vi "ProcessingVehiclesCommandString.vi"(11 "input string":string) -> (3 "output cluster":T1)   [LabVIEW 2013]
panel:
  out "Lane Offset":dbl
  out "Vehicle Id":i32
  out "Time":dbl
  out "Current Distance":dbl
  out "Desired Distance":dbl
  out "Velocity Value":dbl format="%#_13g"
  out "Is Cruise Control":bool
  out "Lane String":string
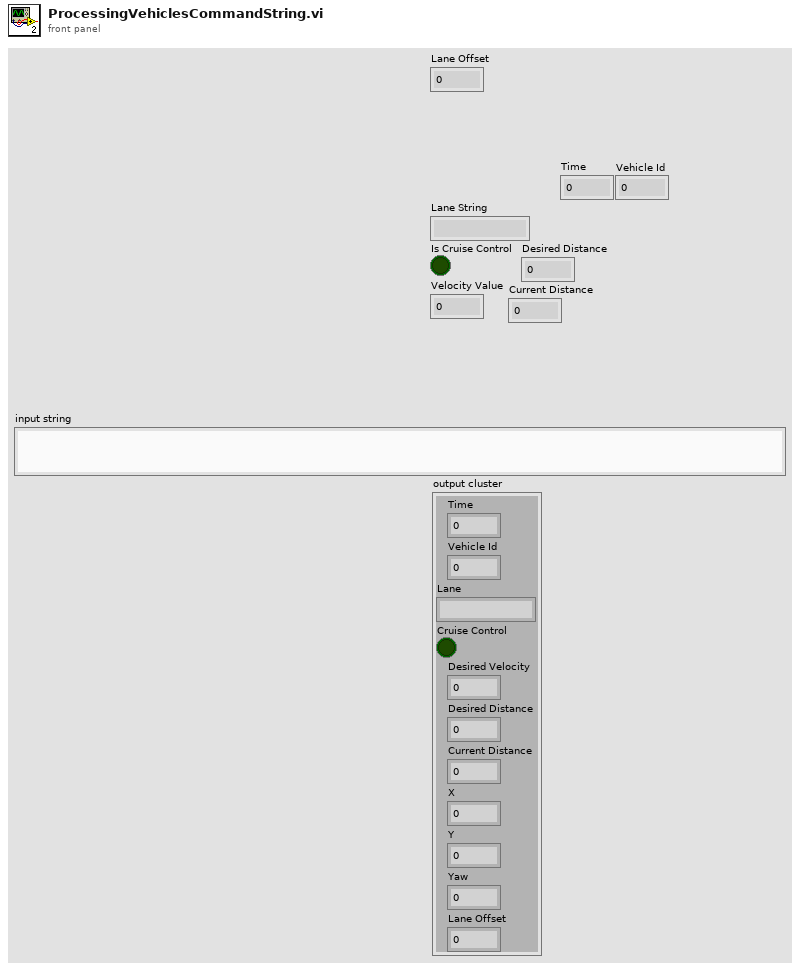
[diagram p1: front panel]
types:
  T1 = cluster{"Time":dbl, "Vehicle Id":i32, "Lane":string, "Cruise Control":bool, "Desired Velocity":dbl, "Desired Distance":dbl, "Current Distance":dbl, "X":dbl, "Y":dbl, "Yaw":dbl, "Lane Offset":dbl}
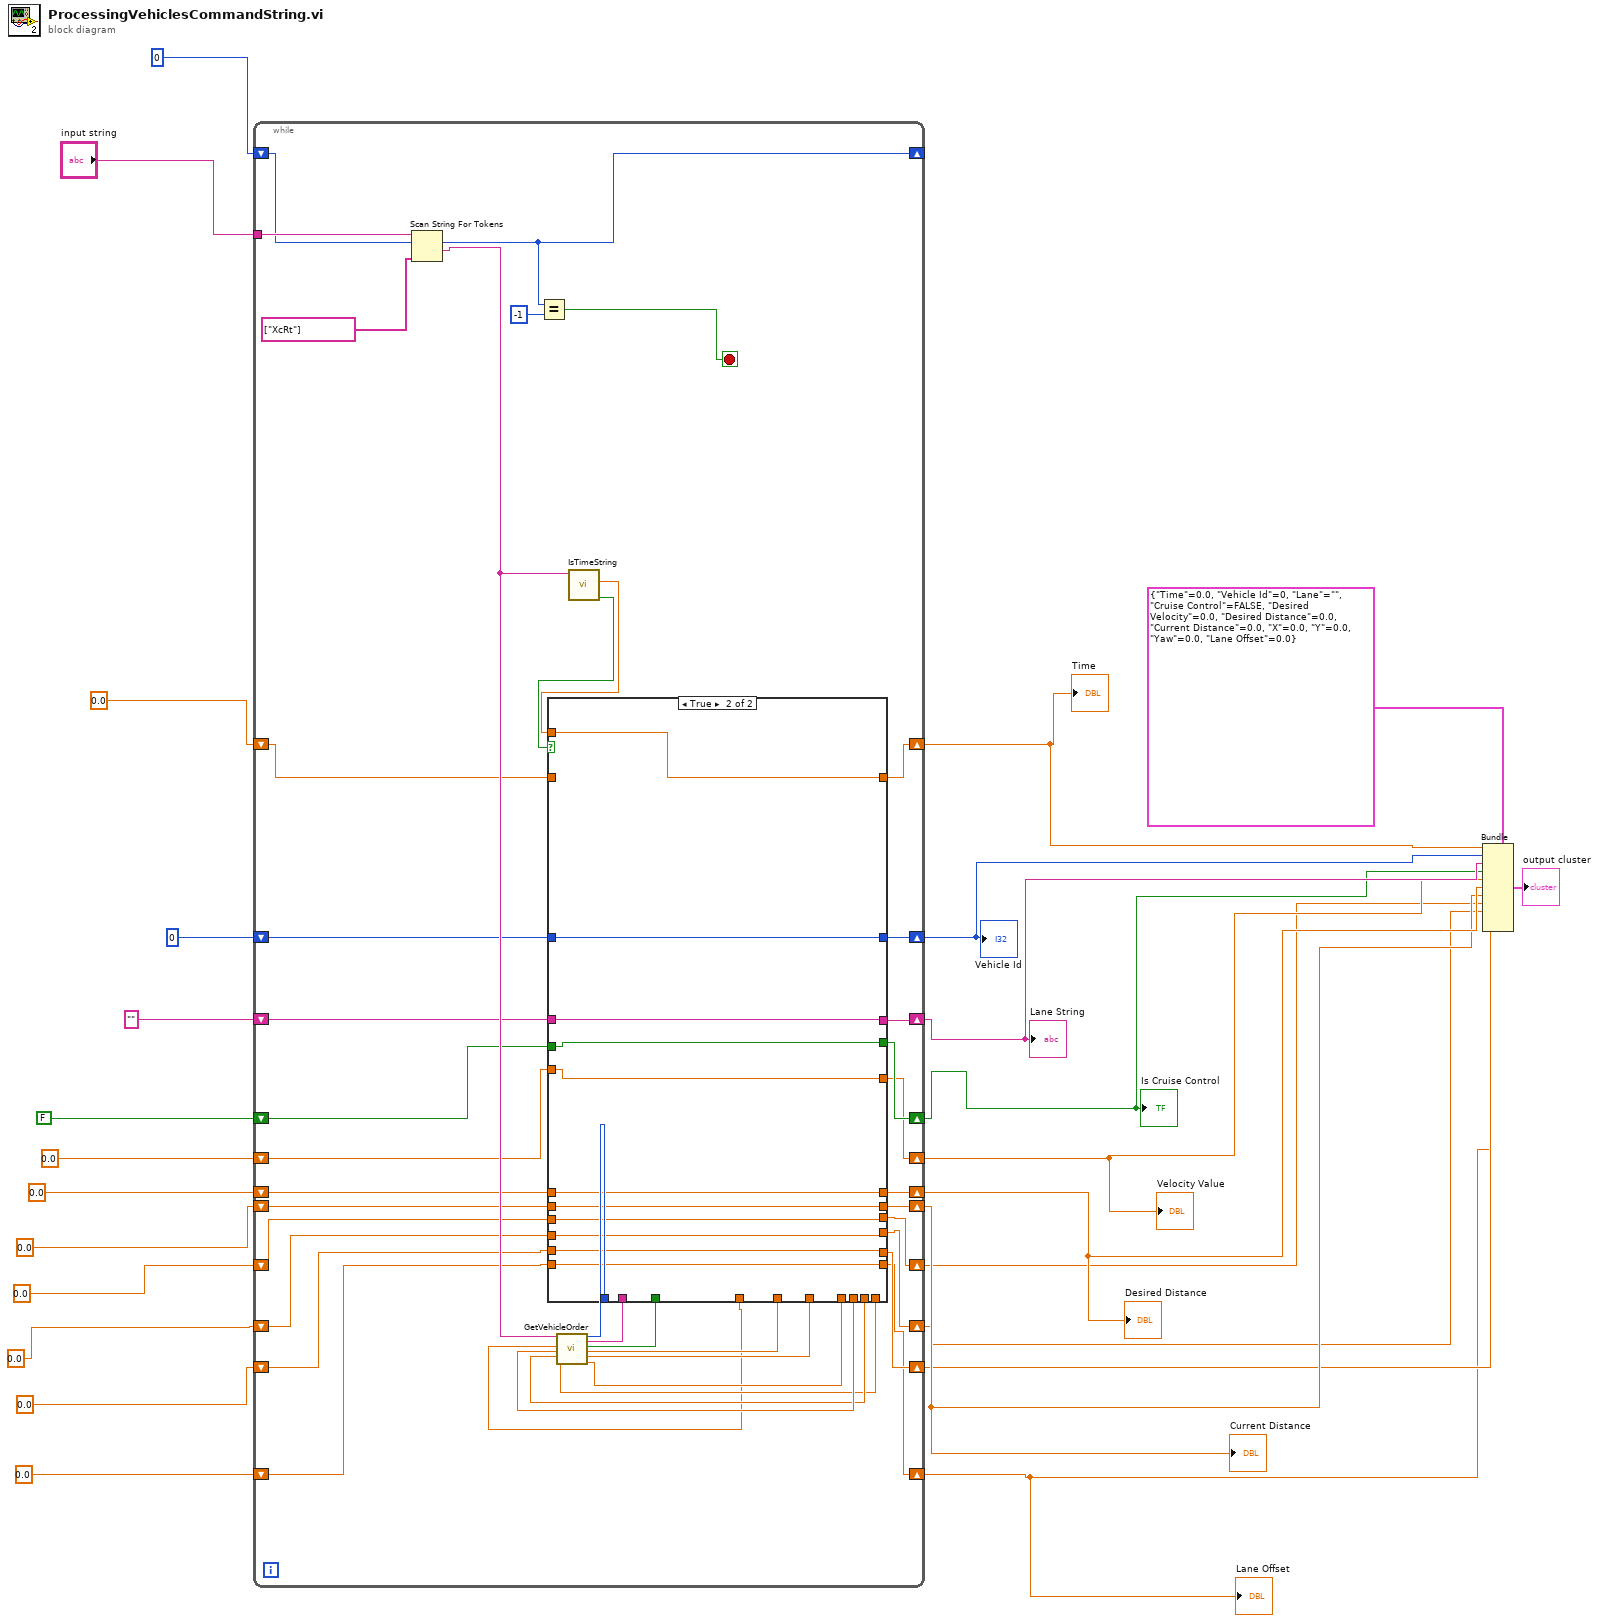
[diagram p0: block diagram]
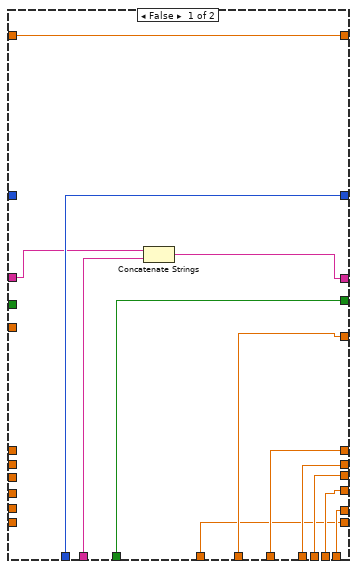
[diagram p2: hidden frame]
diagram:
  n1 = while {
    tunnel: "input string" -> [w67]
    shift-right: [w63] -> _
    shift-left: 0 -> [w64]
    shift-right: [w60] -> w17
    shift-left: 0.0 -> [w59]
    shift-right: [w55] -> w16
    shift-left: 0 -> [w56]
    shift-right: [w52] -> w15
    shift-left: "" -> [w53]
    shift-right: [w48] -> w14
    shift-left: FALSE -> [w50]
    shift-right: [w46] -> w13
    shift-left: 0.0 -> [w47]
    shift-right: [w45] -> w12
    shift-left: 0.0 -> [w44]
    shift-right: [w40] -> w11
    shift-left: 0.0 -> [w39]
    shift-right: [w35] -> w6
    shift-left: 0.0 -> [w38]
    shift-right: [w34] -> w5
    shift-left: 0.0 -> [w37]
    shift-right: [w33] -> w4
    shift-left: 0.0 -> [w36]
    shift-right: [w28] -> w2
    shift-left: 0.0 -> [w29]
    stop <- w65 stop-if-true
    n2 = Scan String For Tokens(6:string[] ["XcRt"] ("delimiters (\\s,\\t,\\r,\\n)"), 8:w64, 9:w67) -> (1:w62:string, 2:w63:i32)  [unwired: 3 in, 2 out]
    n3 = Equal?(x=w63, y=-1) -> (x = y?=w65:bool)
    n4 = call "GetVehicleOrder.vi"("Input String"=w62) -> ("Lane Offset"=w27:dbl, "X"=w32:dbl, "Y"=w31:dbl, "Yaw"=w30:dbl, "Vehicle Id"=w54:i32, "Lane String"=w51:string, "Is Cruise Control"=w49:bool, "Velocity Value"=w43:dbl, "Desired Distance"=w42:dbl, "Current Distance"=w41:dbl)  [unwired: 9 in]
    n5 = call "IsTimeString.vi"("Input String"=w62) -> ("Numeric Value"=w58:dbl, "Is Time String"=w57:bool)  [unwired: 7 in, 1 out]
    n6 = case shown="True" w57 {
      tunnel: [w80 w91] -> w60
      tunnel: w59 -> [w80 _]
      tunnel: w58 -> [_ w91]
      tunnel: w56 -> [_ w90]
      tunnel: [w79 w90] -> w55
      tunnel: w54 -> [w79 _]
      tunnel: [w76 w89] -> w52
      tunnel: w53 -> [w78 w89]
      tunnel: w51 -> [w77 _]
      tunnel: w50 -> [_ w88]
      tunnel: [w75 w88] -> w48
      tunnel: w49 -> [w75 _]
      tunnel: w47 -> [_ w87]
      tunnel: [w74 w87] -> w46
      tunnel: [w73 w86] -> w45
      tunnel: w44 -> [_ w86]
      tunnel: w43 -> [w74 _]
      tunnel: w42 -> [w73 _]
      tunnel: [w72 w85] -> w40
      tunnel: w41 -> [w72 _]
      tunnel: w39 -> [_ w85]
      tunnel: w38 -> [_ w84]
      tunnel: w37 -> [_ w83]
      tunnel: w36 -> [_ w82]
      tunnel: [w71 w84] -> w35
      tunnel: [w70 w83] -> w34
      tunnel: [w69 w82] -> w33
      tunnel: w32 -> [w71 _]
      tunnel: w31 -> [w70 _]
      tunnel: w30 -> [w69 _]
      tunnel: w29 -> [_ w81]
      tunnel: [w68 w81] -> w28
      tunnel: w27 -> [w68 _]
      frame False {
        n7 = Concatenate Strings(w78, w77) -> (w76:string)
      }
      frame True {
      }
    }
  }
  "Time" <- w17
  "Vehicle Id" <- w16
  "Lane String" <- w15
  "Is Cruise Control" <- w14
  "Velocity Value" <- w13
  "Desired Distance" <- w12
  "Current Distance" <- w11
  "Lane Offset" <- w2
  n8 = Bundle(cluster=T1 {"Time"=0.0, "Vehicle Id"=0, "Lane"="", "Cruise Control"=FALSE, "Desired Velocity"=0.0, "Desired Distance"=0.0, "Current Distance"=0.0, "X"=0.0, "Y"=0.0, "Yaw"=0.0, "Lane Offset"=0.0}, "Time"=w17, "Vehicle Id"=w16, "Lane"=w15, "Cruise Control"=w14, "Desired Velocity"=w13, "Desired Distance"=w12, "Current Distance"=w11, "X"=w6, "Y"=w5, "Yaw"=w4, "Lane Offset"=w2) -> (→"output cluster":T1)
